vi "ykgw g.vi"(7 "date in":dbl[](array[numeric])) -> (5 "date out":dbl[](array[numeric]))   [LabVIEW 2019]
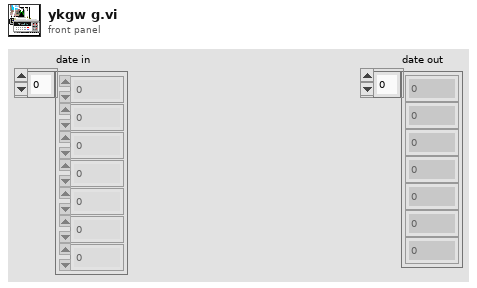
[diagram p1: front panel]
types:
  T1 = cluster{"date in[0]":dbl, "date in[1]":dbl, "date in[2]":dbl, "date in[3]":dbl, "date in[4]":dbl, "date in[5]":dbl, "date in[6]":dbl, "date in[7]":dbl, "date in[8]":dbl}
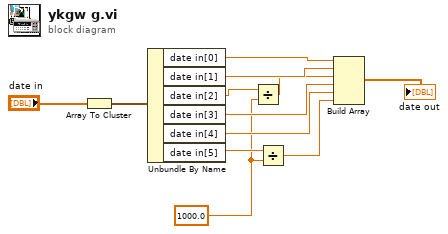
[diagram p0: block diagram]
diagram:
  w2 = 1000.0
  n1 = Array To Cluster(array="date in") -> (cluster=w11:T1)
  n2 = Unbundle By Name(w11) -> ("date in[0]"=w9:dbl, "date in[1]"=w8:dbl, "date in[2]"=w3:dbl, "date in[3]"=w6:dbl, "date in[4]"=w5:dbl, "date in[5]"=w4:dbl)
  n3 = Divide(x=w3, y=w2) -> (x/y=w7:dbl)
  n4 = Divide(x=w4, y=w2) -> (x/y=w1:dbl)
  n5 = Build Array(w9, w8, w7, w6, w5, w1) -> (→"date out":dbl[])
